vi "MicroscopeObjectiveConfigurationWindow.vi"(8 "error in (no error)":errorcluster) -> (0 "error out":errorcluster)   [LabVIEW 2017]
doc: "Use this template to build a VI to use as a subVI."
uses:
  DatabaseContollerGFVenum.ctl
  Objective_cluster.ctl
  <vilib>/addons/Database/_DB Variant To Data/Database Variant To Data.xnode
panel:
  in  "Setup":u16(ring) items=["Gulliver", "Perlman"]
  in  "Cancel Button":bool
  in  "CreateUser Button":bool
  in  "Save Button":bool
  in  "Objectivs ListBox":i32(listbox)
  in  "Description\n(Magnification)":string
  in  "Active Checkbox":bool
  out "Index":i32
  in  "Model":string
  in  "Working\nDistance (mm)":string
  in  "Manufacturer":string
  in  "Microns\nper Pixels":dbl
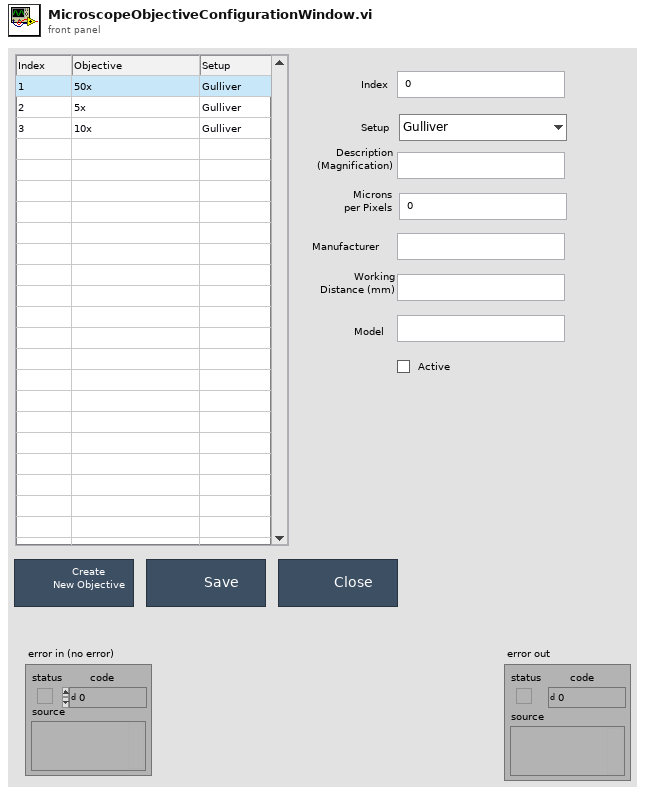
[diagram p1: front panel]
types:
  T1 = typedef "DatabaseContollerGFVenum.ctl" = enum16{"WriteNewUserData!", "Init and Open Database!", "GetAllObjectives!", "GetObjectivesForListBox", "UpdateUserData!", "GetUserData!", "GetUsersAllTable!", "GetTimeDifferencebetweenLastTwoMeasurements!", "Get next Journal Number!", "WriteInJournalTable", "GetNewMeas_dataIndex", "UpdateWithSpectrometerData", "UpdateWithMicroscopeData", "UpdateWithMapScriptData", "UpdateWithmainUIData", "Get Objective Microns/Pixels", "Get User Name!", "Get Next User ID!", "Get Active Users Names!", "Get User Picture!", "Get User Phone Number!", "Get Setup Names!", "Get Active Microscope Objectives!", "Get Experiment Number!", "Get Sample Types!", "Write meas_conf Table", "Write meas_data Table", "GetListOfIndices", "Get Objective Index", "Get last X Journal Entries"}
  T2 = typedef "Objective_cluster.ctl" = cluster{"Index":i32, "Setup":i32, "Description\n(Magnification)":string, "Microns\nper Pixels":dbl, "Manufacturer":string, "Working\nDistance (mm)":string, "Active Checkbox":bool, "Model":string}
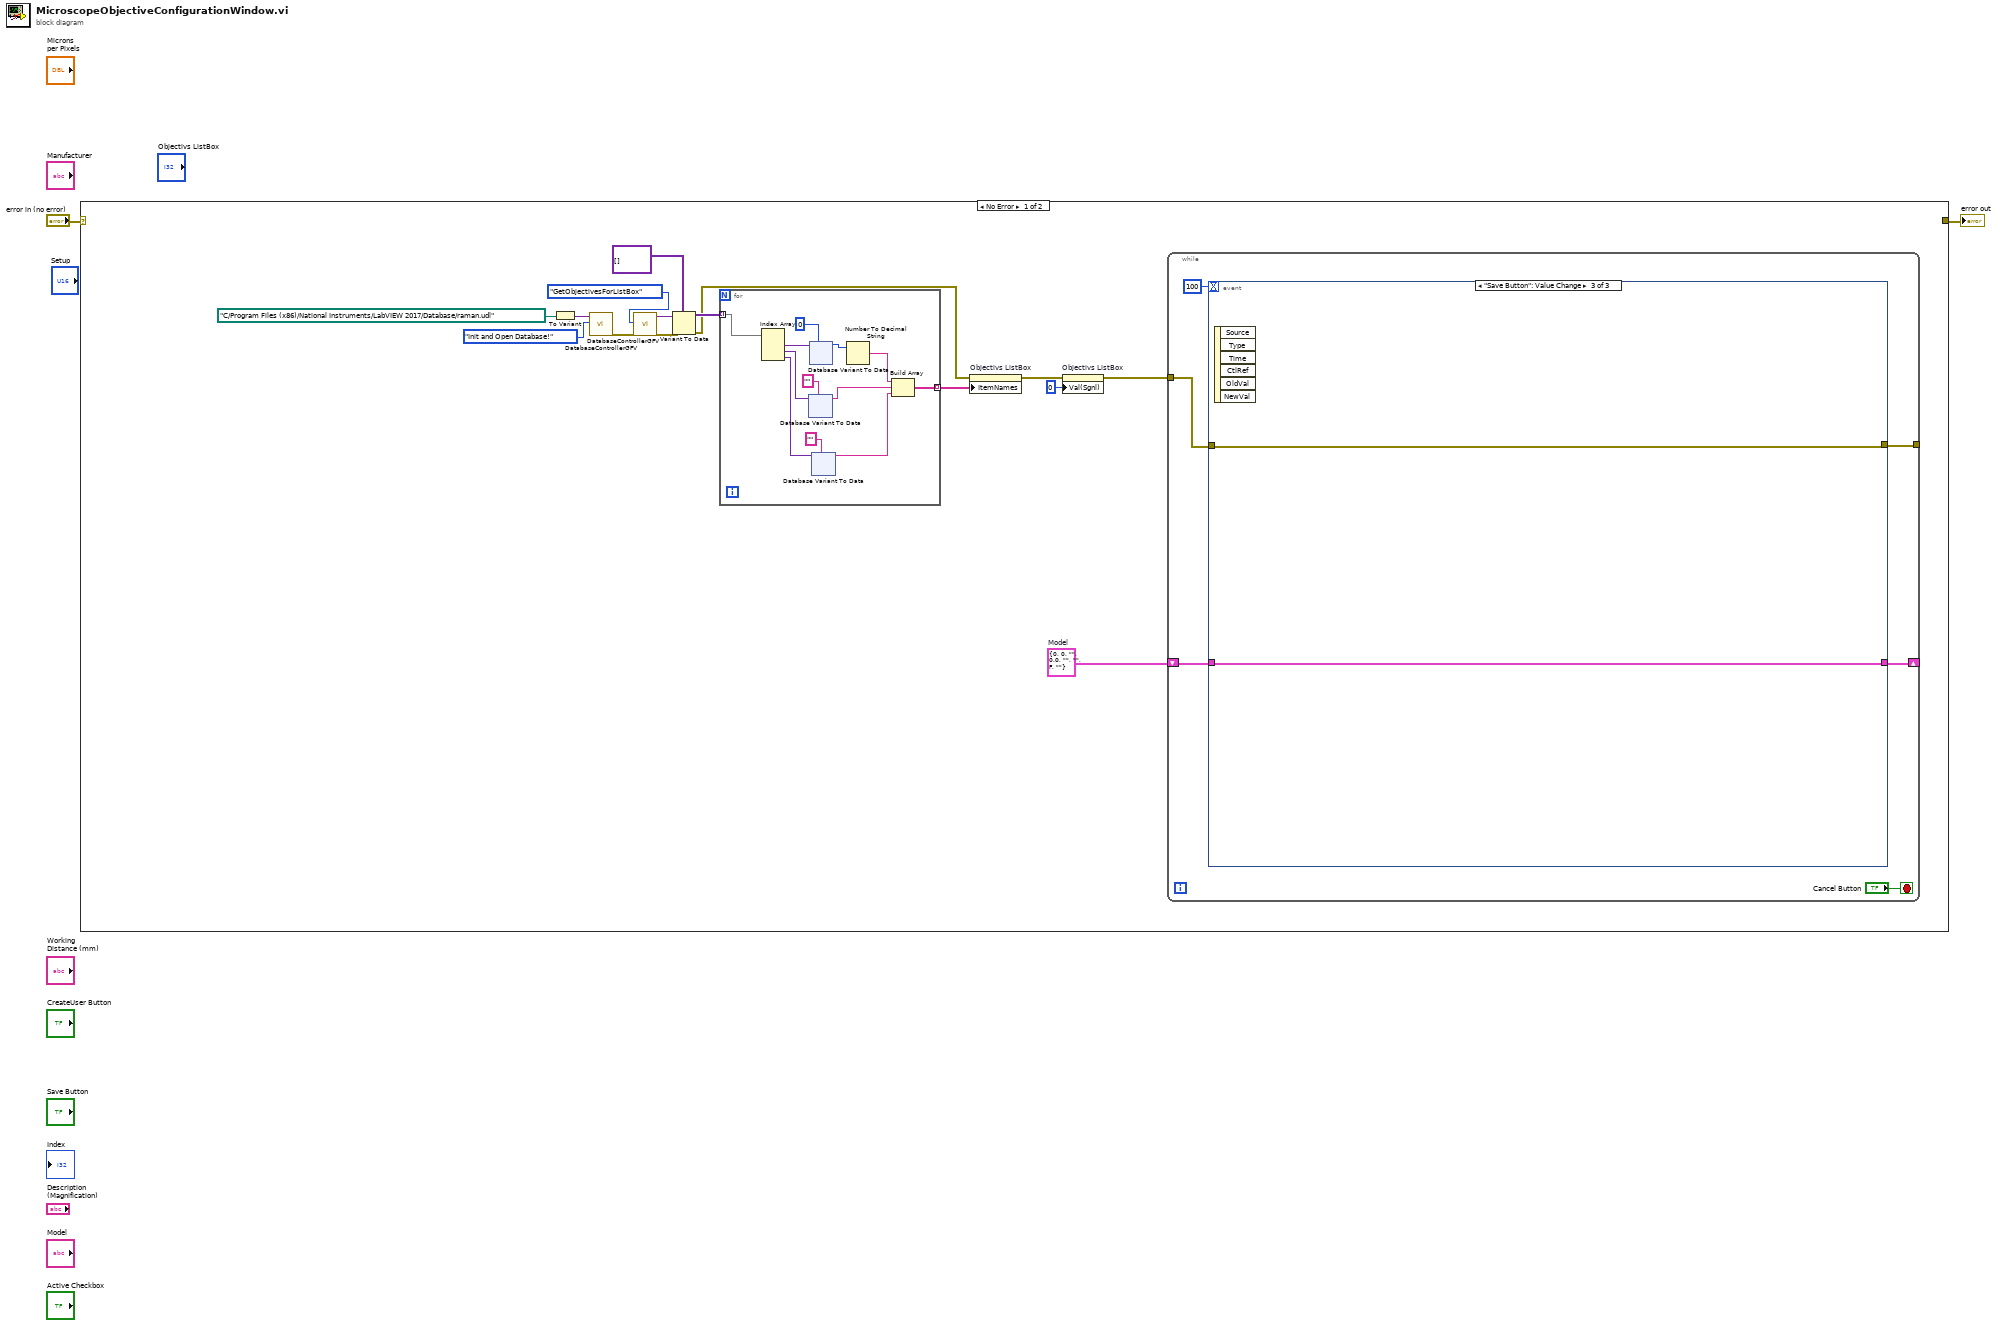
[diagram p0: block diagram]
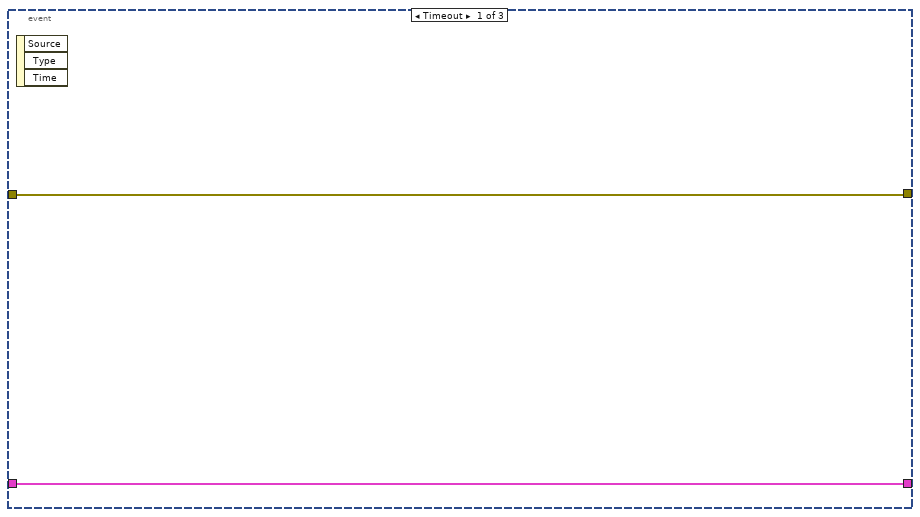
[diagram p2: hidden frame]
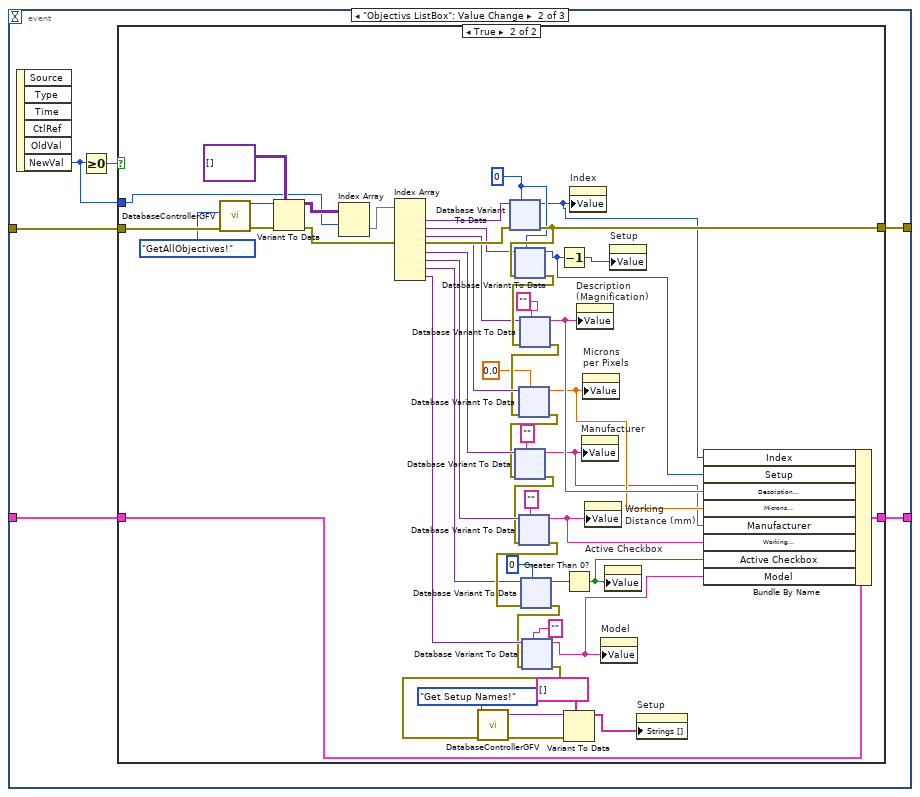
[diagram p3: hidden frame]
diagram:
  n1 = case shown="No Error" "error in (no error)" {
    selector: "error in (no error)" -> [_ w449]
    tunnel: [_ w449] -> w1
    frame No Error {
      w3 = T2 {"Index"=0, "Setup"=0, "Description\n(Magnification)"="", "Microns\nper Pixels"=0.0, "Manufacturer"="", "Working\nDistance (mm)"="", "Active Checkbox"=FALSE, "Model"=""}  # Model
      n2 = To Variant(anything=path "C:/Program Files (x86)/National Instruments/LabVIEW 2017/Database/raman.udl" ("connection information")) -> (Variant=w16:variant)
      n3 = call "DatabaseControllerGFV.vi"("Enum"=DatabaseContollerGFVenum."Init and Open Database!", "Data in"=w16) -> ("error out"=w14:errorcluster)  [unwired: 8 in, 1 out]
      n4 = call "DatabaseControllerGFV.vi"("error in (no error)"=w14, "Enum"=DatabaseContollerGFVenum."GetObjectivesForListBox") -> ("error out"=w13:errorcluster, "Data Out"=w12:variant)  [unwired: 8 in]
      n5 = Variant To Data(error in=w13, type=variant[][] [] ("data"), Variant=w12) -> (data=w9:variant[][], error out=w7:errorcluster)
      n6 = for {
        tunnel: w9 -> [w346] mode=indexing
        tunnel: [w341] -> w8 mode=indexing
        n7 = Index Array(array=w346) -> (element #1=w352:variant, element #2=w350:variant, element #3=w347:variant)  [unwired: 3 in]
        n8 = xnode "Database Variant To Data"("database variant"=w350, "type"="" ("data 2")) -> ("data"=w342:string)  [unwired: 1 in, 1 out]
        n9 = xnode "Database Variant To Data"("database variant"=w352, "type"=0 ("data")) -> ("data"=w345:i32)  [unwired: 1 in, 1 out]
        n10 = xnode "Database Variant To Data"("database variant"=w347, "type"="" ("data 2")) -> ("data"=w343:string)  [unwired: 1 in, 1 out]
        n11 = Number To Decimal String(number=w345) -> (decimal integer string=w344:string)  [unwired: 1 in]
        n12 = Build Array(w344, w342, w343) -> (w341:string[])
      }
      n13 = property on="Objectivs ListBox" class="MCListbox (strict)"(error in=w7, "ItemNames"=w8) -> (error out=w6:errorcluster)  [unwired: 1 in, 1 out]
      n14 = property on="Objectivs ListBox" class="MCListbox (strict)"(error in=w6, "Val(Sgnl)"=0 ("Value (Signaling)")) -> (error out=w5:errorcluster)  [unwired: 1 in, 1 out]
      n15 = while {
        tunnel: w5 -> [w21]
        tunnel: [w20] -> _
        shift-right: [w18] -> _
        shift-left: w3 -> [w19]
        stop <- "Cancel Button" stop-if-true
        n16 = event shown="[2] \"Save Button\": Value Change" {
          selector: _ -> [_ _ _]
          dyn-events: _ -> [_ _ _]
          timeout: 100 -> [_ _ _]
          tunnel: w21 -> [w25 w29 w340]
          tunnel: [w25 w28 w340] -> w20
          tunnel: w19 -> [w24 w27 w339]
          tunnel: [w24 w26 w339] -> w18
          event Timeout {
            n17 = event-data() -> ()  [unwired: 1 in, 3 out]
          }
          event "Objectivs ListBox": Value Change {
            n18 = event-data() -> ("NewVal"=w30:i32)  [unwired: 1 in, 5 out]
            n19 = Greater Or Equal To 0?(x=w30) -> (x >= 0?=w31:bool)
            n20 = case shown="True" w31 {
              tunnel: w30 -> [_ w76]
              tunnel: w29 -> [w33 w82]
              tunnel: [w33 w72] -> w28
              tunnel: w27 -> [w32 w43]
              tunnel: [w32 w34] -> w26
              frame False {
              }
              frame True {
                w70 = 0 ("data")
                n21 = call "DatabaseControllerGFV.vi"("error in (no error)"=w82, "Enum"=DatabaseContollerGFVenum."GetAllObjectives!") -> ("error out"=w78:errorcluster, "Data Out"=w79:variant)  [unwired: 8 in]
                n22 = Variant To Data(error in=w78, type=variant[][] [] ("data"), Variant=w79) -> (data=w77:variant[][], error out=w73:errorcluster)
                n23 = Index Array(array=w77, index (row)=w76) -> (element=w75:variant[])  [unwired: 1 in]
                n24 = Index Array(array=w75) -> (element #1=w74:variant, element #2=w71:variant, element #3=w68:variant, element #4=w66:variant, element #5=w62:variant, element #6=w59:variant, element #7=w56:variant, element #8=w54:variant)  [unwired: 8 in]
                n25 = xnode "Database Variant To Data"("database variant"=w74, "error in (no error)"=w73, "type"=w70) -> ("data"=w42:i32, "error out"=w72:errorcluster)
                n26 = xnode "Database Variant To Data"("database variant"=w71, "error in (no error)"=w72, "type"=w70) -> ("data"=w41:i32, "error out"=w69:errorcluster)
                n27 = xnode "Database Variant To Data"("database variant"=w68, "error in (no error)"=w69, "type"="" ("Description\n(Magnification)")) -> ("data"=w40:string, "error out"=w65:errorcluster)
                n28 = xnode "Database Variant To Data"("database variant"=w66, "error in (no error)"=w65, "type"=0.0 ("Microns\nper Pixels")) -> ("data"=w39:dbl, "error out"=w61:errorcluster)
                n29 = xnode "Database Variant To Data"("database variant"=w62, "error in (no error)"=w61, "type"="" ("Description\n(Magnification)")) -> ("data"=w38:string, "error out"=w58:errorcluster)
                n30 = xnode "Database Variant To Data"("database variant"=w59, "error in (no error)"=w58, "type"="" ("Description\n(Magnification)")) -> ("data"=w37:string, "error out"=w57:errorcluster)
                n31 = xnode "Database Variant To Data"("database variant"=w56, "error in (no error)"=w57, "type"=0 ("data")) -> ("data"=w51:i32, "error out"=w53:errorcluster)
                n32 = xnode "Database Variant To Data"("database variant"=w54, "error in (no error)"=w53, "type"="" ("Description\n(Magnification)")) -> ("data"=w35:string, "error out"=w46:errorcluster)
                n33 = call "DatabaseControllerGFV.vi"("error in (no error)"=w46, "Enum"=DatabaseContollerGFVenum."Get Setup Names!") -> ("error out"=w50:errorcluster, "Data Out"=w49:variant)  [unwired: 8 in]
                n34 = Decrement(x=w41) -> (x-1=w44:i32)
                n35 = Greater Than 0?(x=w51) -> (x > 0?=w36:bool)
                n36 = Variant To Data(error in=w50, type=string[] [], Variant=w49) -> (data=w45:string[])  [unwired: 1 out]
                n37 = property on="Index" class="DigNum (strict)"("Value"=w42) -> ()  [unwired: 2 in, 2 out]
                n38 = property on="Description\n(Magnification)" class="Str"("Value"=w40) -> ()  [unwired: 2 in, 2 out]
                n39 = property on="Manufacturer" class="Str"("Value"=w38) -> ()  [unwired: 2 in, 2 out]
                n40 = property on="Microns\nper Pixels" class="DigNum (strict)"("Value"=w39) -> ()  [unwired: 2 in, 2 out]
                n41 = property on="Working\nDistance (mm)" class="Str"("Value"=w37) -> ()  [unwired: 2 in, 2 out]
                n42 = property on="Model" class="Str"("Value"=w35) -> ()  [unwired: 2 in, 2 out]
                n43 = property on="Active Checkbox" class="Bool (strict)"("Value"=w36) -> ()  [unwired: 2 in, 2 out]
                n44 = property on="Setup" class="Ring (strict)"("Value"=w44) -> ()  [unwired: 2 in, 2 out]
                n45 = property on="Setup" class="Ring (strict)"("Strings []"=w45) -> ()  [unwired: 2 in, 2 out]
                n46 = Bundle By Name(cluster=w43, "Index"=w42, "Setup"=w41, "Description\n(Magnification)"=w40, "Microns\nper Pixels"=w39, "Manufacturer"=w38, "Working\nDistance (mm)"=w37, "Active Checkbox"=w36, "Model"=w35) -> (w34:T2)
              }
            }
          }
          event "Save Button": Value Change {
            n47 = event-data() -> ()  [unwired: 1 in, 6 out]
          }
        }
      }
    }
    frame Error {
    }
  }
  "error out" <- w1
